vi "Transcriptor LabVIEW to C code Step 0 Create Definitions.vi"(8 "error in":errorcluster, 11 "Diagram in":refnum<vi>) -> (0 "error out":errorcluster, 3 "structure definitions cluster":T1)   [LabVIEW 2014]
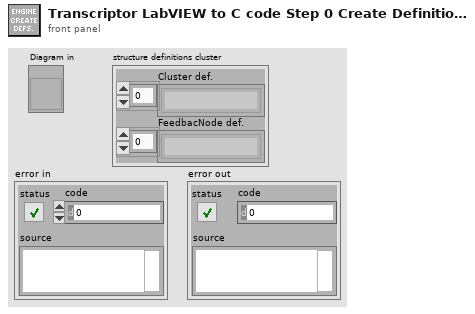
[diagram p1: front panel]
types:
  T1 = cluster{"Cluster def.":string[], "FeedbacNode def.":string[]}
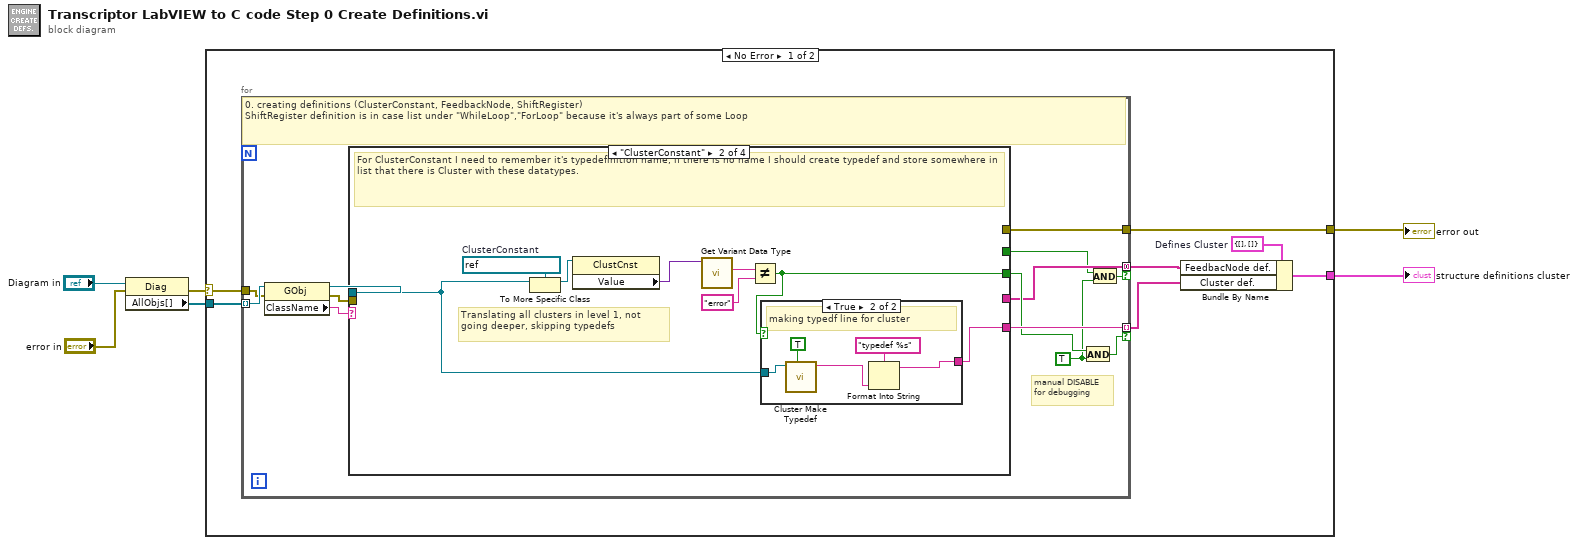
[diagram p0: block diagram]
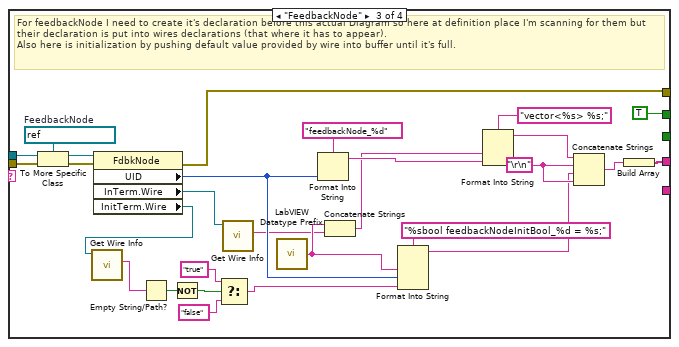
[diagram p4: hidden frame]
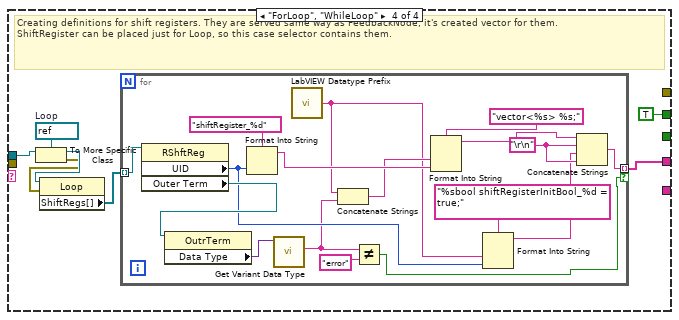
[diagram p5: hidden frame]
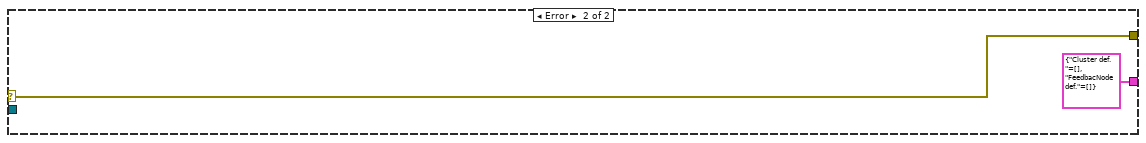
[diagram p6: hidden frame]
diagram:
  n1 = property class="Diag"(reference="Diagram in", error in="error in") -> (error out=w2:errorcluster, "AllObjs[]"=w5:refnum<vi>[])  [unwired: 1 out]
  n2 = case shown="No Error" w2 {
    selector: w2 -> [w8 w92]
    tunnel: [w13 T1 {"Cluster def."=[], "FeedbacNode def."=[]} ("Defines Cluster")] -> w6
    tunnel: w5 -> [w9 _]
    tunnel: [w7 w92] -> w1
    frame No Error {
      w10 = T1 {"Cluster def."=[], "FeedbacNode def."=[]}  # Defines Cluster
      n3 = for {
        tunnel: w9 -> [w26] mode=indexing
        tunnel: [w23] -> w11 mode=indexing if=w21
        tunnel: [w20] -> w12 mode=concatenating if=w19
        tunnel: w8 -> [w16]
        tunnel: [w14] -> w7
        w17 = TRUE
        # "manual DISABLE\nfor debugging"
        # "0. creating definitions (ClusterConstant, FeedbackNode, ShiftRegister)\nShiftRegister definition is in case list under \"WhileLoop\",\"ForLoop\" because it's always part of some Loop"
        n4 = property class="GObj"(reference=w26, error in=w16) -> (reference out=w24:refnum<vi>, error out=w15:errorcluster, "ClassName"=w25:string)
        n5 = case shown="\"ClusterConstant\"" w25 {
          tunnel: w24 -> [_ w29 w62 w70]
          tunnel: [_ w27 _ _] -> w23
          tunnel: [_ w30 _ _] -> w22
          tunnel: [_ _ w50 w68] -> w20
          tunnel: [_ _ TRUE TRUE] -> w18
          tunnel: w15 -> [_ _ w41 _]
          tunnel: [_ _ w40 _] -> w14
          frame Default {
            # "If wire is not wired to anything from what I have to read value, output is default Variant value (hope that is empty Variant), and there will be just wire declaration without assignement in generated code."
          }
          frame "ClusterConstant" {
            w31 = refnum<vi> refnum  # ClusterConstant
            # "Translating all clusters in level 1, not going deeper, skipping typedefs"
            # "For ClusterConstant I need to remember it's typedefinition name, if there is no name I should create typedef and store somewhere in list that there is Cluster with these datatypes."
            n6 = To More Specific Class(target class=w31, reference=w29) -> (specific class reference=w28:refnum<vi>)  [unwired: 1 in, 1 out]
            n7 = property on="Property Node" class="ClustCnst"(reference=w28) -> ("Value"=w34:variant)  [unwired: 1 in, 2 out]
            n8 = call "Get Variant Data Type.vi"("Variant in"=w34) -> ("first data type"=w33:string)  [unwired: 9 in, 1 out]
            n9 = Not Equal?(x=w33, y="error") -> (x != y?=w30:bool)
            n10 = case shown="True" w30 {
              tunnel: w29 -> [_ w39]
              tunnel: [_ w35] -> w27
              frame False {
              }
              frame True {
                # "making typedf line for cluster"
                n11 = call "Cluster Make Typedef.vi"("skip first typedef?"=TRUE, "ClusterConstant refnum in"=w39) -> ("String"=w36:string)  [unwired: 9 in]
                n12 = Format Into String(format string="typedef %s", w36) -> (resulting string=w35:string)  [unwired: 2 in, 1 out]
              }
            }
          }
          frame "FeedbackNode" {
            w56 = "\r\n"
            w67 = refnum<vi> refnum  # FeedbackNode
            # "For feedbackNode I need to create it's declaration before this actual Diagram so here at definition place I'm scanning for them but their declaration is put into wires declarations (that where it has to appear).\nAlso here is initialization by pushing default value provided by wire into buffer until it's full."
            n13 = To More Specific Class(target class=w67, reference=w62, error in=w41) -> (specific class reference=w66:refnum<vi>, error out=w65:errorcluster)
            n14 = property class="FdbkNode"(reference=w66, error in=w65) -> (error out=w40:errorcluster, "UID"=w57:i32, "InTerm.Wire"=w54:refnum<vi>, "InitTerm.Wire"=w43:refnum<vi>)  [unwired: 1 out]
            n15 = call "Get Wire Info.vi"("Wire"=w43) -> ("wire datatype"=w42:string)  [unwired: 9 in, 1 out]
            n16 = Empty String/Path?(string/path=w42) -> (empty?=w48:bool)
            n17 = Not(x=w48) -> (.not. x?=w47:bool)
            n18 = Select(t="true" ("format string"), s=w47, f="false" ("format string")) -> (s? t:f=w44:string)
            n19 = call "Get Wire Info.vi"("Wire"=w54) -> ("wire datatype"=w49:string)  [unwired: 9 in, 1 out]
            n20 = call "LabVIEW Datatype Prefix.vi"() -> ("datatype prefix"=w52:string)
            n21 = Format Into String(format string="feedbackNode_%d", w57) -> (resulting string=w59:string)  [unwired: 2 in, 1 out]
            n22 = Concatenate Strings(w52, w49) -> (w53:string)
            n23 = Format Into String(format string="%sbool feedbackNodeInitBool_%d = %s;", w52, w57, w44) -> (resulting string=w55:string)  [unwired: 2 in, 1 out]
            n24 = Format Into String(format string="vector<%s> %s;", w53, w59) -> (resulting string=w60:string)  [unwired: 2 in, 1 out]
            n25 = Concatenate Strings(w60, w56, w55, w56) -> (w51:string)
            n26 = Build Array(w51) -> (w50:string[])
          }
          frame "ForLoop", "WhileLoop" {
            w73 = refnum<vi> refnum  # Loop
            # "Creating definitions for shift registers. They are served same way as FeedbackNode, it's created vector for them.\nShiftRegister can be placed just for Loop, so this case selector contains them."
            n27 = To More Specific Class(target class=w73, reference=w70) -> (specific class reference=w72:refnum<vi>, error out=w71:errorcluster)  [unwired: 1 in]
            n28 = property class="Loop"(reference=w72, error in=w71) -> ("ShiftRegs[]"=w69:refnum<vi>[])  [unwired: 2 out]
            n29 = for {
              tunnel: w69 -> [w91] mode=indexing
              tunnel: [w80] -> w68 mode=indexing if=w77
              w83 = "\r\n"
              n30 = property class="RShftReg"(reference=w91) -> ("UID"=w79:i32, "Outer Term"=w88:refnum<vi>)  [unwired: 1 in, 2 out]
              n31 = property class="OutrTerm"(reference=w88) -> ("Data Type"=w76:variant)  [unwired: 1 in, 2 out]
              n32 = Format Into String(format string="shiftRegister_%d", w79) -> (resulting string=w89:string)  [unwired: 2 in, 1 out]
              n33 = call "Get Variant Data Type.vi"("Variant in"=w76) -> ("first data type"=w75:string)  [unwired: 9 in, 1 out]
              n34 = call "LabVIEW Datatype Prefix.vi"() -> ("datatype prefix"=w84:string)
              n35 = Concatenate Strings(w84, w75) -> (w86:string)
              n36 = Not Equal?(x=w75, y="error") -> (x != y?=w77:bool)
              n37 = Format Into String(format string="vector<%s> %s;", w86, w89) -> (resulting string=w82:string)  [unwired: 2 in, 1 out]
              n38 = Format Into String(format string="%sbool shiftRegisterInitBool_%d = true;", w84, w79) -> (resulting string=w81:string)  [unwired: 2 in, 1 out]
              n39 = Concatenate Strings(w82, w83, w81, w83) -> (w80:string)
            }
          }
        }
        n40 = And(x=w22, y=w17) -> (x .and. y?=w21:bool)
        n41 = And(x=w18, y=w17) -> (x .and. y?=w19:bool)
      }
      n42 = Bundle By Name(cluster=w10, "FeedbacNode def."=w12, "Cluster def."=w11) -> (w13:T1)
    }
    frame Error {
    }
  }
  "structure definitions cluster" <- w6
  "error out" <- w1
